vi "Set Panes to Origins.vi"(8 "error in (no error)":errorcluster, 11 "IViewManager In":refnum<class "IViewManager.lvclass">) -> (0 "error out":errorcluster, 3 "IViewManager Out":refnum<class "IViewManager.lvclass">)   [LabVIEW 2020, in "IViewManager.lvlib" / "IViewManager.lvclass"]
doc: "<License>\nCopyright © 2017 Composed Systems, LLC | All rights reserved\nwww.composed.io\n\nAuthor: Ethan Stern <ethan.stern@composed.io>\n\nThis software is provided \"AS IS\" WITHOUT WARRANTIES, either express or implied, AND IS FOR EDUCATIONAL PURPOSES ONLY.\n</License>"
uses:
  <vilib>/gpm_packages/@cs/mva-viewable/Source/IViewManager/IViewManager/IViewManager.lvclass
  <vilib>/gpm_packages/@cs/mva-viewable/Source/IViewManager/IViewManager/IViewManager.lvclass/IViewManager.ctl
  <vilib>/ActorFramework/Message Enqueuer/Message Enqueuer.lvclass/Message Enqueuer.ctl
  <vilib>/ActorFramework/Message Enqueuer/Enqueue.vi
  <vilib>/gpm_packages/@cs/mva-viewable/Source/IViewable/IViewable Messages/Set Panes to Origins Msg/Set Panes to Origins Msg.lvclass
  C:/Program Files/National Instruments/LabVIEW 2020/vi.lib/ActorFramework/Message/Message.lvclass
  <vilib>/ActorFramework/Message Priority Queue/Priority Enqueue.vi
  <vilib>/gpm_packages/@cs/mva-viewable/Source/IViewable/IViewable/IViewable.lvclass
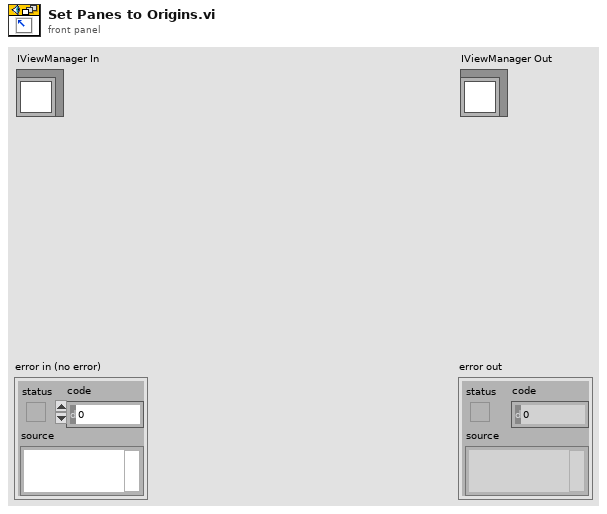
[diagram p1: front panel]
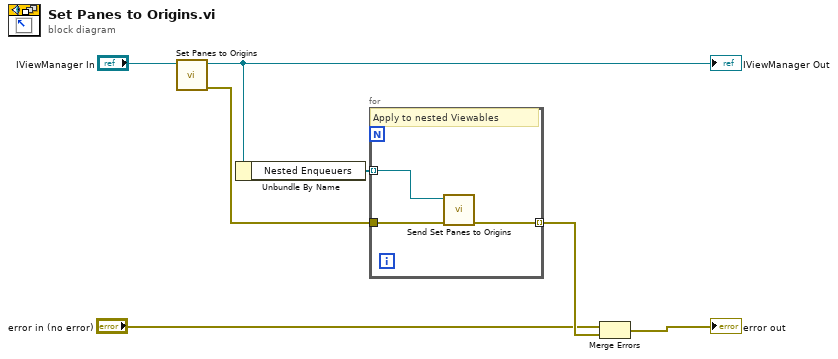
[diagram p0: block diagram]
diagram:
  n1 = call-parent "Set Panes to Origins.vi"("IViewable In"="IViewManager In") -> ("error out"=w7:errorcluster, "IViewable Out"=w5:refnum<class "IViewManager.lvclass">)  [unwired: 9 in]
  "IViewManager Out" <- w5
  n2 = Unbundle By Name(w5) -> ("Nested Enqueuers"=w3:refnum<class "Message Enqueuer.lvclass">[])
  n3 = for {
    tunnel: w3 -> [w10] mode=indexing
    tunnel: w7 -> [w9]
    tunnel: [w8] -> w4 mode=indexing
    # "Apply to nested Viewables"
    n4 = call <vilib>:"Send Set Panes to Origins.vi"("error in (no error)"=w9, "Message Enqueuer"=w10) -> ("error out"=w8:errorcluster)  [unwired: 8 in, 1 out]
  }
  n5 = Merge Errors("error in (no error)", w4) -> (→"error out":errorcluster)
